vi "FTW-Actor-Initialize.vi"(0 "FTW Actor Instance Type":refnum<class "FTW-ActorInstance.lvclass">, 5 "Initialization Job Sequence":string, 7 "Actor Instance Configuration":string, 11 "error in":errorcluster) -> (4 "FTW Actor Instance":refnum<class "FTW-ActorInstance.lvclass">, 8 "Event Refnums":T1, 15 "error out":errorcluster)   [LabVIEW 2015, in "FTW-ActorInstance.lvclass"]
uses:
  FTW-ActorInstance.lvclass
  Message/Request/FTW-Message-IncomingRequest.lvclass
  Message/Base/FTW-Message.lvclass
  FTW-Actor-FrameworkEvent.ctl
  FTW-ActorInstance.lvclass/FTW-ActorInstance.ctl
  JSON/core/FTW-JSON-Core-EncodingFlags.vi
  JSON/FTW-JSON-Parse.vi
  Reflection/FTW-Reflection-Type.vi
  CodeGen/JSON Deserialize/FTW-JSON-Core-GetFlattenedValue.vi
  CodeGen/JSON Deserialize/FTW-JSON-Deserialize.xnode
  JobSequencer/FTW-JobSequencer.lvclass
panel:
  # "Inputs"
  # "Outputs"
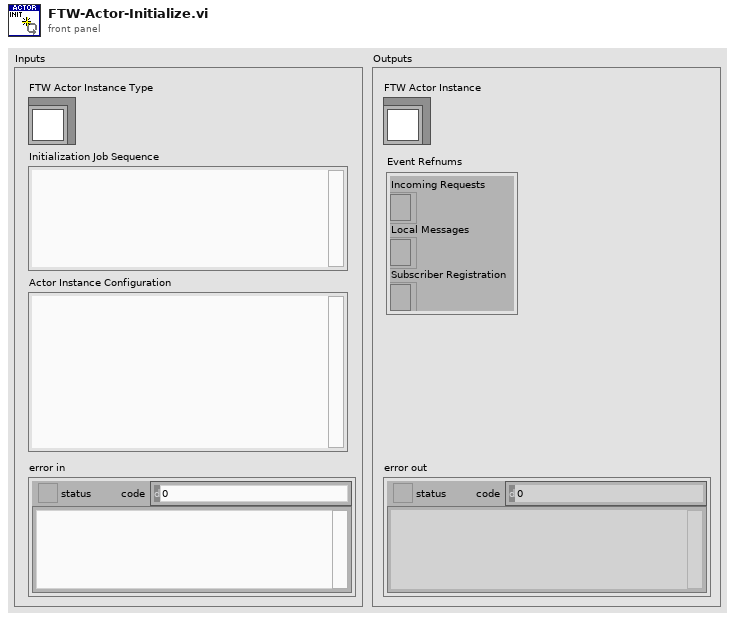
[diagram p1: front panel]
types:
  T1 = cluster{"Incoming Requests":refnum<event-registration>, "Local Messages":refnum<event-registration>, "Subscriber Registration":refnum<event-registration>}
  T2 = typedef "FTW-ActorInstance.lvclass/FTW-Actor-FrameworkEvent.ctl" = enum16{"Instance Initializing", "Instance Constructed", "Instance Initialized", "Instance Initialization Failed", "Instance Job", "Instance Handle Request", "Instance Shutting Down", "Instance Destroyed"}
  T3 = cluster{"Identity":string, "DebugShowPanel":bool}
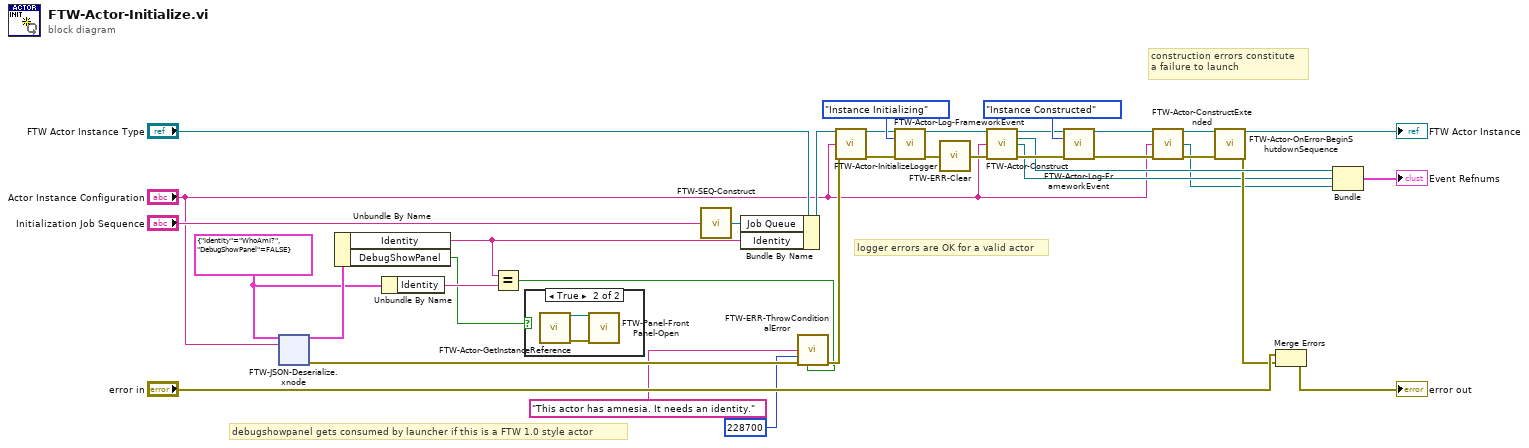
[diagram p0: block diagram]
diagram:
  w16 = T3 {"Identity"="WhoAmI?", "DebugShowPanel"=FALSE}
  # "debugshowpanel gets consumed by launcher if this is a FTW 1.0 style actor"
  # "logger errors are OK for a valid actor"
  # "construction errors constitute\na failure to launch"
  n1 = xnode "FTW-JSON-Deserialize.xnode"("Type and Defaults"=w16, "JSON String"="Actor Instance Configuration") -> ("Values"=w17:T3, "error out"=w30:errorcluster)  [unwired: 1 in]
  n2 = Unbundle By Name(w17) -> ("Identity"=w9:string, "DebugShowPanel"=w8:bool)
  n3 = Unbundle By Name(w16) -> ("Identity"=w10:string)
  n4 = Equal?(x=w9, y=w10) -> (x = y?=w14:bool)
  n5 = case shown="True" w8 {
    frame False {
    }
    frame True {
      n6 = call "FTW-Actor-GetInstanceReference.vi"() -> ("Actor Refnum"=w38:refnum<vi>, "error out"=w37:errorcluster)  [unwired: 14 in]
      n7 = call "FTW-Panel-FrontPanel-Open.vi"("error in"=w37, "VI Ref"=w38) -> ()  [unwired: 8 in, 2 out]
    }
  }
  n8 = call "FTW-SEQ-Construct.vi"("Initial Sequence"="Initialization Job Sequence") -> ("FTW Job Sequencer"=w32:refnum<class "FTW-JobSequencer.lvclass">)
  n9 = Bundle By Name(cluster="FTW Actor Instance Type", "Job Queue"=w32, "Identity"=w9) -> (w27:refnum<class "FTW-ActorInstance.lvclass">)
  n10 = call "FTW-ERR-ThrowConditionalError.vi"("Error Message"="This actor has amnesia. It needs an identity." ("Warning Message"), "Error Code"=228700, "error in"=w30, "Throw Error?"=w14) -> ("error out"=w15:errorcluster)  [unwired: 11 in]
  n11 = call-dynamic "FTW-Actor-InitializeLogger.vi"("FTW Actor Instance Type"=w27, "Actor Instance Configuration"="Actor Instance Configuration", "error in"=w15) -> ("FTW Actor Instance"=w26:refnum<class "FTW-ActorInstance.lvclass">, "error out"=w33:errorcluster)  [unwired: 11 in]
  n12 = call "FTW-Actor-Log-FrameworkEvent.vi"("FTW Actor Instance"=w26, "Framework Event"=FTW-Actor-FrameworkEvent."Instance Initializing", "error in"=w33) -> ("FTW Actor Instance out"=w24:refnum<class "FTW-ActorInstance.lvclass">, "error out"=w34:errorcluster)  [unwired: 11 in]
  n13 = call "FTW-ERR-Clear.vi"("error to snuff"=w34) -> ("no error"=w31:errorcluster)
  n14 = call-dynamic "FTW-Actor-Construct.vi"("FTW Actor Instance Type"=w24, "Actor Instance Configuration"="Actor Instance Configuration", "error in"=w31) -> ("FTW Actor Instance"=w23:refnum<class "FTW-ActorInstance.lvclass">, "Incoming Requests"=w20:refnum<event-registration>, "Local Messages"=w6:refnum<event-registration>, "error out"=w25:errorcluster)  [unwired: 9 in]
  n15 = call "FTW-Actor-Log-FrameworkEvent.vi"("FTW Actor Instance"=w23, "Framework Event"=FTW-Actor-FrameworkEvent."Instance Constructed", "error in"=w25) -> ("FTW Actor Instance out"=w4:refnum<class "FTW-ActorInstance.lvclass">, "error out"=w11:errorcluster)  [unwired: 11 in]
  n16 = call-dynamic "FTW-Actor-ConstructExtended.vi"("FTW Actor Instance Type"=w4, "Actor Instance Configuration"="Actor Instance Configuration", "error in"=w11) -> ("FTW Actor Instance"=w3:refnum<class "FTW-ActorInstance.lvclass">, "Subscriber Registration"=w1:refnum<event-registration>, "error out"=w5:errorcluster)  [unwired: 10 in]
  n17 = call-dynamic "FTW-Actor-OnError-BeginShutdownSequence.vi"("FTW Actor Instance"=w3, "error in"=w5) -> ("FTW Actor Instance out"=→"FTW Actor Instance":refnum<class "FTW-ActorInstance.lvclass">, "error out"=w19:errorcluster)  [unwired: 12 in]
  n18 = Merge Errors("error in", w19) -> (→"error out":errorcluster)
  n19 = Bundle("Incoming Requests"=w20, "Local Messages"=w6, "Subscriber Registration"=w1) -> (→"Event Refnums":T1)  [unwired: 1 in]
